vi "Destructor.vi"(8 "error in":errorcluster, 11 "IntegerMeasureLimit":refnum<class "IntegerMeasureLimit.lvclass">) -> (0 "error out":errorcluster)   [LabVIEW 2021, in "ProligentXMLGenerator.lvlib" / "IntegerMeasureLimit.lvclass"]
uses:
  IntegerMeasureLimit.lvclass
  IntegerMeasureLimit.lvclass/IntegerMeasureLimit.ctl
  MeasureLimit/MeasureLimit.lvclass
  RangeMeasureLimit/RangeMeasureLimit.lvclass
  C:/Projects/proligent-xml-generator-labview/src/ProligentXMLGenerator/Measure/RangeMeasureLimit/RangeMeasureLimit.lvclass
  C:/Projects/proligent-xml-generator-labview/src/ProligentXMLGenerator/Measure/MeasureLimit/MeasureLimit.lvclass
  C:/Projects/proligent-xml-generator-labview/src/ProligentXMLGenerator/Measure/IntegerMeasureLimit/IntegerMeasureLimit.lvclass
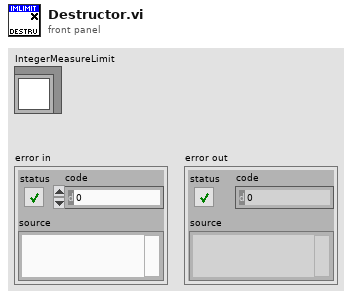
[diagram p1: front panel]
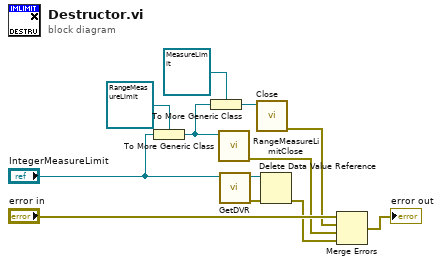
[diagram p0: block diagram]
diagram:
  n1 = To More Generic Class(target class=refnum<class "RangeMeasureLimit.lvclass"> refnum ("ProligentResultProcessor:RangeMeasureLimit"), reference="IntegerMeasureLimit") -> (generic class reference=w4:refnum<class "RangeMeasureLimit.lvclass">)
  n2 = To More Generic Class(target class=refnum<class "MeasureLimit.lvclass"> refnum ("ProligentResultProcessor:MeasureLimit"), reference=w4) -> (generic class reference=w5:refnum<class "MeasureLimit.lvclass">)
  n3 = call "RangeMeasureLimitClose.vi"("RangeMeasureLimit"=w4) -> ("error out"=w1:errorcluster)  [unwired: 10 in]
  n4 = call "GetDVR.vi"("IntegerMeasureLimit"="IntegerMeasureLimit") -> ("error out"=w9:errorcluster, "DVRReference"=w10:refnum<data-value>)  [unwired: 9 in]
  n5 = call "Close.vi"("MeasureLimit"=w5) -> ("error out"=w2:errorcluster)  [unwired: 10 in]
  n6 = Delete Data Value Reference(data value reference=w10, error in=w9) -> (error out=w8:errorcluster)  [unwired: 1 out]
  n7 = Merge Errors("error in", w2, w1, w8) -> (→"error out":errorcluster)
